vi "ImageData.vi"(2 "bytes to read":i32=2111488, 3 "timeout ms":i32=10000, 4 "command":string="controller.GetImageData()") -> (0 "unsigned byte array":u8[](array[numeric]), 1 "Error":bool=TRUE)   [LabVIEW 2014]
uses:
  globals/AzCamGlobals.vi
panel:
  out "error out":errorcluster={"status"=TRUE, "code"=56, "source"="TCP Read in ImageData.vi->GetImageData.vi->AzCamTool.vi"}
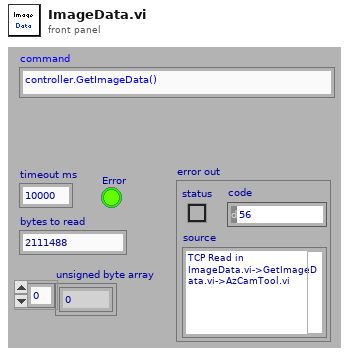
[diagram p1: front panel]
types:
  T1 = enum16{"Standard", "Buffered", "CRLF", "Immediate"}
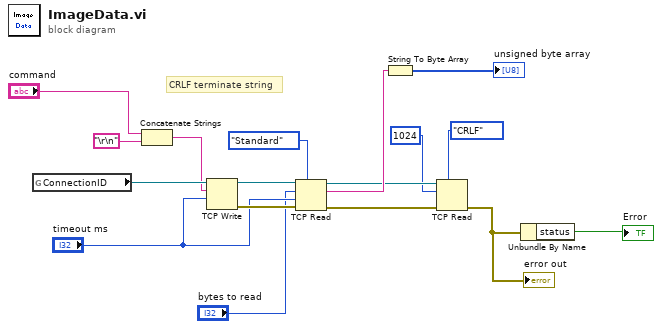
[diagram p0: block diagram]
diagram:
  # "CRLF terminate string"
  n1 = global read "AzCamGlobals.vi" "ConnectionID"() -> (w11:refnum<k5>)
  n2 = Concatenate Strings("command", "\r\n") -> (w9:string)
  n3 = TCP Write(connection ID=w11, data in=w9, 9:"timeout ms") -> (connection ID out=w15:refnum<k5>, error out=w14:errorcluster)  [unwired: 1 in, 1 out]
  n4 = TCP Read(connection ID=w15, bytes to read="bytes to read", error in (no error)=w14, 7:T1."Standard" ("mode (standard)"), 9:"timeout ms") -> (connection ID out=w5:refnum<k5>, data out=w7:string, error out=w2:errorcluster)
  n5 = String To Byte Array(string=w7) -> (unsigned byte array=→"unsigned byte array":u8[])
  n6 = TCP Read(connection ID=w5, bytes to read=1024, error in (no error)=w2, 7:T1."CRLF" ("mode (standard)")) -> (error out=w1:errorcluster)  [unwired: 1 in, 2 out]
  "error out" <- w1
  n7 = Unbundle By Name(w1) -> ("status"=→"Error":bool)
